vi "Update Active VI.vi"(6 "VIWindow":i32, 9 "VIName":string, 10 "Application in":refnum<vi>, 11 "Data in":T1) -> (3 "Data out":T1)   [LabVIEW 2020, in "Peek Window.lvlib"]
uses:
  Peek Window.lvlib
  Active VI Cluster.ctl
  EHL Data Cluster.ctl
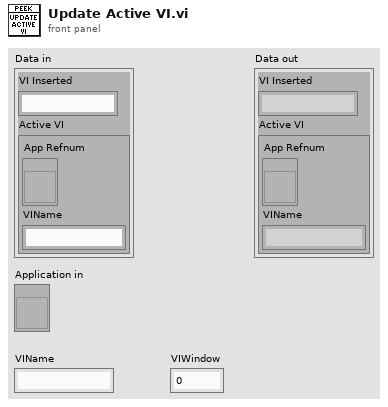
[diagram p1: front panel]
types:
  T1 = typedef "Peek Window.lvlib/EHL Data Cluster.ctl" = cluster{"VI Inserted":string, "Active VI":T2}
  T2 = typedef "Peek Window.lvlib/Active VI Cluster.ctl" = cluster{"App Refnum":refnum<vi>, "VIName":string}
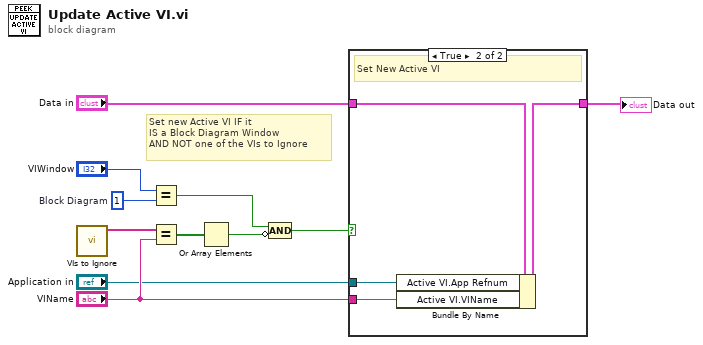
[diagram p0: block diagram]
diagram:
  w3 = 1  # Block Diagram
  # "Set new Active VI IF it\nIS a Block Diagram Window\nAND NOT one of the VIs to Ignore"
  n1 = call "VIs to Ignore.vi"() -> ("VIs to Ignore"=w10:string[])  [unwired: 11 in]
  n2 = Equal?(x="VIWindow", y=w3) -> (x = y?=w2:bool)
  n3 = Equal?(x=w10, y="VIName") -> (x = y?=w6:bool[])
  n4 = Or Array Elements(Boolean array=w6) -> (logical OR=w8:bool)
  n5 = Compound Arithmetic op=AND(w2, invert w8) -> (w5:bool)
  n6 = case shown="True" w5 {
    tunnel: "Application in" -> [_ w16]
    tunnel: "VIName" -> [_ w15]
    tunnel: "Data in" -> [w12 w14]
    tunnel: [w12 w13] -> w1
    frame False {
      # "Continue with previous Active VI"
    }
    frame True {
      # "Set New Active VI"
      n7 = Bundle By Name(cluster=w14, "Active VI.App Refnum"=w16, "Active VI.VIName"=w15) -> (w13:T1)
    }
  }
  "Data out" <- w1
